vi "TDMS2TDMProperties.vi"(8 "error in (no error)":errorcluster, 9 "property names":string[](array[string]), 10 "property values":variant[](array[variant]), 11 "new storage refnum":refnum<k20>) -> (0 "error out":errorcluster, 3 "new storage refnum out":refnum<k20>)   [LabVIEW 2020]
doc: "This VI reads in a list of TDMS properties as variant data. It decodes the original datatype of the variant data and creates TDM properties for a given channel or channel group of that datatype. If an unsupported datatype is used, the data is coerced and the coercion is logged."
uses:
  <vilib>/Utility/tdmsutil.llb/TDMS2TDMNameType.ctl
  <vilib>/Platform/storage/Storage.llb/__savePropInt32.vi
  <vilib>/Utility/tdmsutil.llb/TDMS2TDMLogDataConversion.vi
  <vilib>/Platform/storage/Storage.llb/__savePropInt16.vi
  <vilib>/Platform/storage/Storage.llb/__savePropUInt8.vi
  <vilib>/Platform/storage/Storage.llb/__savePropFloat64.vi
  <vilib>/Platform/storage/Storage.llb/__savePropFloat32.vi
  <vilib>/Platform/storage/Storage.llb/__savePropString.vi
  <vilib>/Platform/storage/Storage.llb/__savePropTime.vi
  <vilib>/Utility/Data Type/NI_Data Type.lvlib
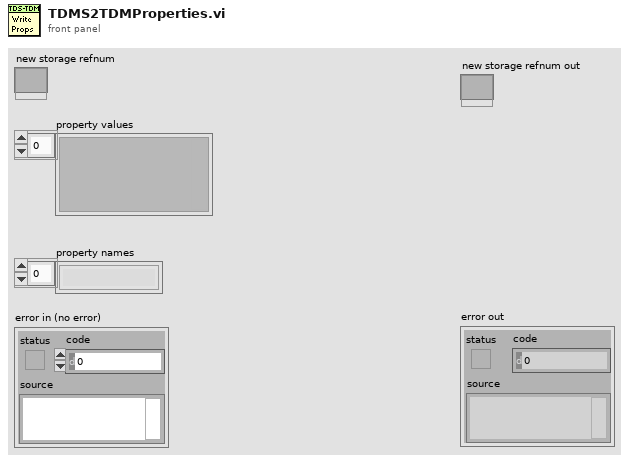
[diagram p1: front panel]
types:
  T1 = typedef "TDMS2TDMNameType.ctl" = enum16{"Channel", "Property"}
  T2 = typedef "NI_Data Type.lvlib/Data Type.ctl" = enum8{"Invalid Type", "Void", "I8", "I16", "I32", "I64", "U8", "U16", "U32", "U64", "Single Float", "Double Float", "Extended Float", "Single Complex", "Double Complex", "Extended Complex", "Enum U8", "Enum U16", "Enum U32", "Enum U64", "Single Float With Unit", "Double Float With Unit", "Extended Float With Unit", "Single Complex with Unit", "Double Complex with Unit", "Extended Complex with Unit", "Boolean", "String", "Path", "Picture", "Tag", "Array", "Cluster", "Variant", "LV Variant", "Waveform", "Timestamp", "Digital Waveform", "Digital Data", "ExpressData", "Refnum", "External Data", "VI", "Poly VI", "LabVIEW Class Instance", "Fixed Point", "Set Collection", "Map Collection"}
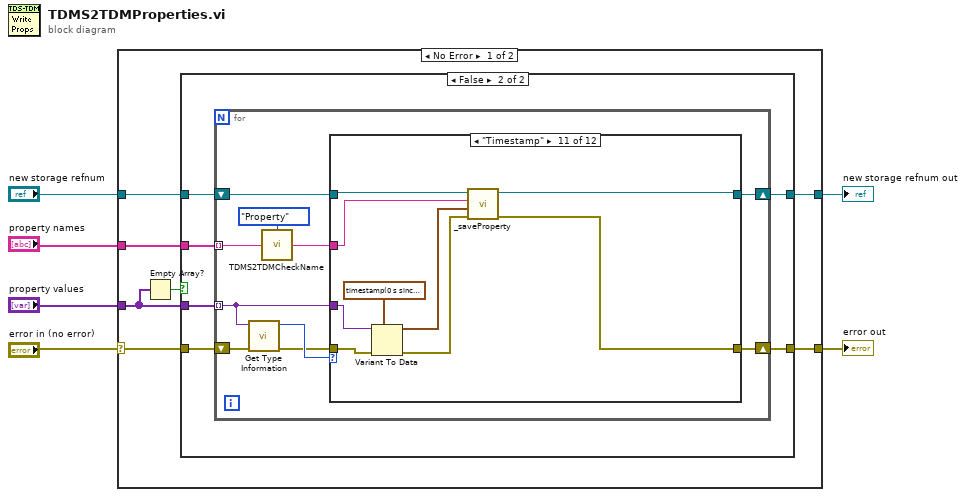
[diagram p0: block diagram]
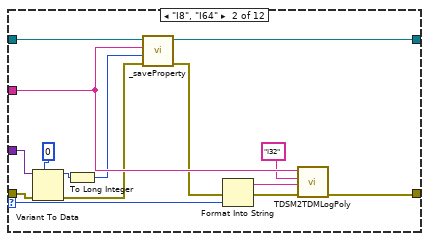
[diagram p4: hidden frame]
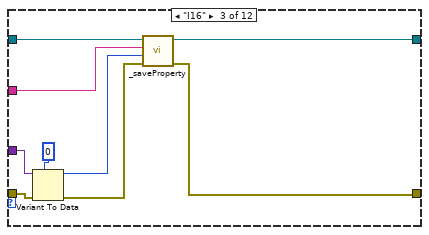
[diagram p5: hidden frame]
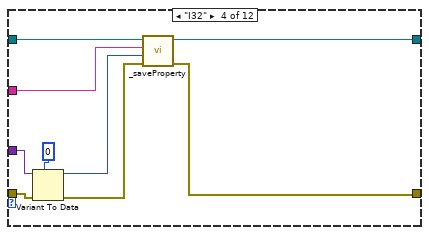
[diagram p6: hidden frame]
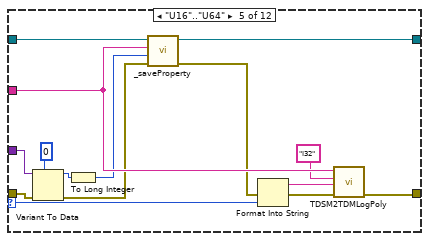
[diagram p7: hidden frame]
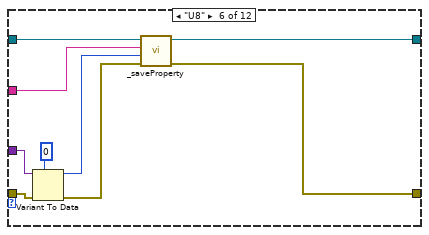
[diagram p8: hidden frame]
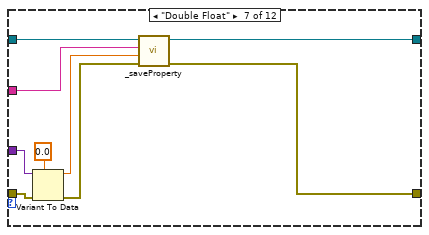
[diagram p9: hidden frame]
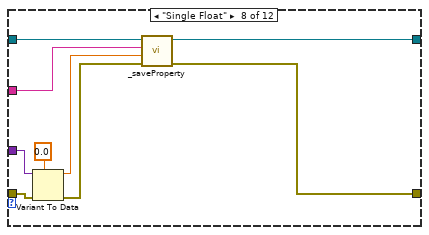
[diagram p10: hidden frame]
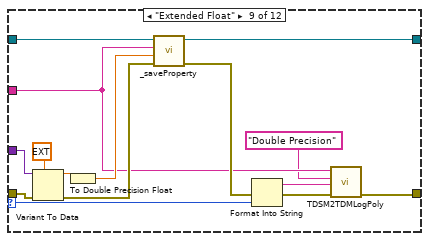
[diagram p11: hidden frame]
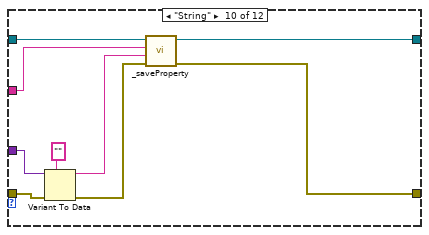
[diagram p12: hidden frame]
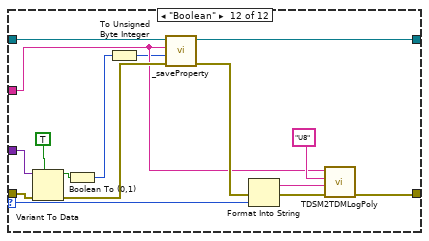
[diagram p13: hidden frame]
diagram:
  n1 = case shown="No Error" "error in (no error)" {
    selector: "error in (no error)" -> [w7 w158]
    tunnel: "property names" -> [w13 _]
    tunnel: "property values" -> [w12 _]
    tunnel: "new storage refnum" -> [w10 w159]
    tunnel: [w9 w159] -> w3
    tunnel: [w8 w158] -> w2
    frame No Error {
      n2 = Empty Array?(array=w12) -> (empty?=w11:bool)
      n3 = case shown="False" w11 {
        tunnel: w13 -> [_ w21]
        tunnel: w12 -> [_ w20]
        tunnel: w10 -> [w15 w19]
        tunnel: [w15 w18] -> w9
        tunnel: w7 -> [w14 w17]
        tunnel: [w14 w16] -> w8
        frame True {
        }
        frame False {
          n4 = for {
            tunnel: w20 -> [w30] mode=indexing
            tunnel: w21 -> [w24] mode=indexing
            shift-right: [w28] -> w18
            shift-left: w19 -> [w29]
            shift-right: [w25] -> w16
            shift-left: w17 -> [w27]
            n5 = call <vilib>:"Get Type Information.vi"("error in (no error)"=w27, "variant"=w30) -> ("error out"=w26:errorcluster, "type"=w31:T2)  [unwired: 5 in, 3 out]
            n6 = call <vilib>:"TDMS2TDMCheckName.vi"("Name Type"=TDMS2TDMNameType."Property", "Name"=w24) -> ("Name Out"=w23:string)  [unwired: 13 in]
            n7 = case shown="\"Timestamp\"" w31 {
              selector: w31 -> [_ w39 _ _ w71 _ _ _ w114 _ _ w143]
              tunnel: w30 -> [_ w47 w56 w65 w80 w90 w99 w108 w123 w132 w141 w156]
              tunnel: w29 -> [w33 w42 w52 w61 w75 w85 w97 w106 w119 w129 w137 w151]
              tunnel: [w33 w43 w53 w62 w76 w87 w96 w105 w118 w128 w135 w152] -> w28
              tunnel: w23 -> [_ w48 w57 w66 w81 w84 w94 w103 w111 w126 w136 w145]
              tunnel: w26 -> [w32 w45 w54 w63 w77 w88 w91 w100 w121 w130 w139 w153]
              tunnel: [w32 w37 w50 w59 w69 w86 w95 w104 w112 w127 w133 w144] -> w25
              frame "Void", Default {
              }
              frame "I8", "I64" {
                n8 = Variant To Data(error in=w45, type=i64 0 ("offset (0)"), Variant=w47) -> (data=w44:i64, error out=w40:errorcluster)
                n9 = To Long Integer(number=w44) -> (32bit integer=w41:i32)
                n10 = call-poly <vilib>:"_saveProperty.vi"("error in (no error)"=w40, "Value"=w41, "Property name"=w48, "storage refnum"=w42) -> ("error out"=w38:errorcluster, "dup storage refnum"=w43:refnum<k20>)  [unwired: 6 in]
                n11 = Format Into String(error in=w38, w39) -> (resulting string=w35:string, error out=w36:errorcluster)  [unwired: 2 in]
                n12 = call-poly <vilib>:"TDSM2TDMLogPoly.vi"("error in (no error)"=w36, "Original Datatype"=w35, "New Datatype"="I32", "Channel Name"=w48) -> ("error out"=w37:errorcluster)  [unwired: 7 in]
              }
              frame "I16" {
                n13 = Variant To Data(error in=w54, type=i16 0 ("offset (0)"), Variant=w56) -> (data=w49:i16, error out=w51:errorcluster)
                n14 = call-poly <vilib>:"_saveProperty.vi"("error in (no error)"=w51, "Value"=w49, "Property name"=w57, "storage refnum"=w52) -> ("error out"=w50:errorcluster, "dup storage refnum"=w53:refnum<k20>)  [unwired: 6 in]
              }
              frame "I32" {
                n15 = Variant To Data(error in=w63, type=0 ("offset (0)"), Variant=w65) -> (data=w58:i32, error out=w60:errorcluster)
                n16 = call-poly <vilib>:"_saveProperty.vi"("error in (no error)"=w60, "Value"=w58, "Property name"=w66, "storage refnum"=w61) -> ("error out"=w59:errorcluster, "dup storage refnum"=w62:refnum<k20>)  [unwired: 6 in]
              }
              frame "U16".."U64" {
                n17 = Variant To Data(error in=w77, type=u64 0 ("offset (0)"), Variant=w80) -> (data=w78:u64, error out=w73:errorcluster)
                n18 = To Long Integer(number=w78) -> (32bit integer=w74:i32)
                n19 = call-poly <vilib>:"_saveProperty.vi"("error in (no error)"=w73, "Value"=w74, "Property name"=w81, "storage refnum"=w75) -> ("error out"=w72:errorcluster, "dup storage refnum"=w76:refnum<k20>)  [unwired: 6 in]
                n20 = Format Into String(error in=w72, w71) -> (resulting string=w68:string, error out=w70:errorcluster)  [unwired: 2 in]
                n21 = call-poly <vilib>:"TDSM2TDMLogPoly.vi"("error in (no error)"=w70, "Original Datatype"=w68, "New Datatype"="I32", "Channel Name"=w81) -> ("error out"=w69:errorcluster)  [unwired: 7 in]
              }
              frame "U8" {
                n22 = Variant To Data(error in=w88, type=u8 0 ("offset (0)"), Variant=w90) -> (data=w82:u8, error out=w83:errorcluster)
                n23 = call-poly <vilib>:"_saveProperty.vi"("error in (no error)"=w83, "Value"=w82, "Property name"=w84, "storage refnum"=w85) -> ("error out"=w86:errorcluster, "dup storage refnum"=w87:refnum<k20>)  [unwired: 6 in]
              }
              frame "Double Float" {
                n24 = Variant To Data(error in=w91, type=0.0 ("offset (0)"), Variant=w99) -> (data=w93:dbl, error out=w92:errorcluster)
                n25 = call-poly <vilib>:"_saveProperty.vi"("error in (no error)"=w92, "Value"=w93, "Property name"=w94, "storage refnum"=w97) -> ("error out"=w95:errorcluster, "dup storage refnum"=w96:refnum<k20>)  [unwired: 6 in]
              }
              frame "Single Float" {
                n26 = Variant To Data(error in=w100, type=sgl 0.0 ("offset (0)"), Variant=w108) -> (data=w102:sgl, error out=w101:errorcluster)
                n27 = call-poly <vilib>:"_saveProperty.vi"("error in (no error)"=w101, "Value"=w102, "Property name"=w103, "storage refnum"=w106) -> ("error out"=w104:errorcluster, "dup storage refnum"=w105:refnum<k20>)  [unwired: 6 in]
              }
              frame "Extended Float" {
                n28 = Variant To Data(error in=w121, type=ext 0.0 ("offset (0)"), Variant=w123) -> (data=w120:ext, error out=w116:errorcluster)
                n29 = To Double Precision Float(number=w120) -> (double precision float=w117:dbl)
                n30 = call-poly <vilib>:"_saveProperty.vi"("error in (no error)"=w116, "Value"=w117, "Property name"=w111, "storage refnum"=w119) -> ("error out"=w115:errorcluster, "dup storage refnum"=w118:refnum<k20>)  [unwired: 6 in]
                n31 = Format Into String(error in=w115, w114) -> (resulting string=w110:string, error out=w113:errorcluster)  [unwired: 2 in]
                n32 = call-poly <vilib>:"TDSM2TDMLogPoly.vi"("error in (no error)"=w113, "Original Datatype"=w110, "New Datatype"="Double Precision", "Channel Name"=w111) -> ("error out"=w112:errorcluster)  [unwired: 7 in]
              }
              frame "String" {
                n33 = Variant To Data(error in=w130, type="" ("offset (0)"), Variant=w132) -> (data=w125:string, error out=w124:errorcluster)
                n34 = call-poly <vilib>:"_saveProperty.vi"("error in (no error)"=w124, "Value"=w125, "Property name"=w126, "storage refnum"=w129) -> ("error out"=w127:errorcluster, "dup storage refnum"=w128:refnum<k20>)  [unwired: 6 in]
              }
              frame "Timestamp" {
                n35 = Variant To Data(error in=w139, type=timestamp(0 s since 1904-01-01), Variant=w141) -> (data=w138:timestamp, error out=w134:errorcluster)
                n36 = call-poly <vilib>:"_saveProperty.vi"("error in (no error)"=w134, "Value"=w138, "Property name"=w136, "storage refnum"=w137) -> ("error out"=w133:errorcluster, "dup storage refnum"=w135:refnum<k20>)  [unwired: 6 in]
              }
              frame "Boolean" {
                n37 = Variant To Data(error in=w153, type=TRUE, Variant=w156) -> (data=w154:bool, error out=w149:errorcluster)
                n38 = Boolean To (0,1)(Boolean=w154) -> (0, 1=w150:i16)
                n39 = To Unsigned Byte Integer(number=w150) -> (unsigned 8bit integer=w142:u8)
                n40 = call-poly <vilib>:"_saveProperty.vi"("error in (no error)"=w149, "Value"=w142, "Property name"=w145, "storage refnum"=w151) -> ("error out"=w148:errorcluster, "dup storage refnum"=w152:refnum<k20>)  [unwired: 6 in]
                n41 = Format Into String(error in=w148, w143) -> (resulting string=w146:string, error out=w147:errorcluster)  [unwired: 2 in]
                n42 = call-poly <vilib>:"TDSM2TDMLogPoly.vi"("error in (no error)"=w147, "Original Datatype"=w146, "New Datatype"="U8", "Channel Name"=w145) -> ("error out"=w144:errorcluster)  [unwired: 7 in]
              }
            }
          }
        }
      }
    }
    frame Error {
    }
  }
  "new storage refnum out" <- w3
  "error out" <- w2
